vi "Get User Filename and Path.vi"(8 "error in (no error)":errorcluster) -> (0 "error out":errorcluster, 2 "TXT File Path":path, 3 "CSV File Path":path)   [LabVIEW 2021]
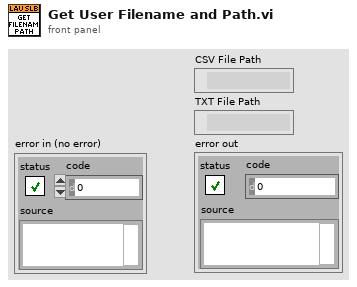
[diagram p1: front panel]
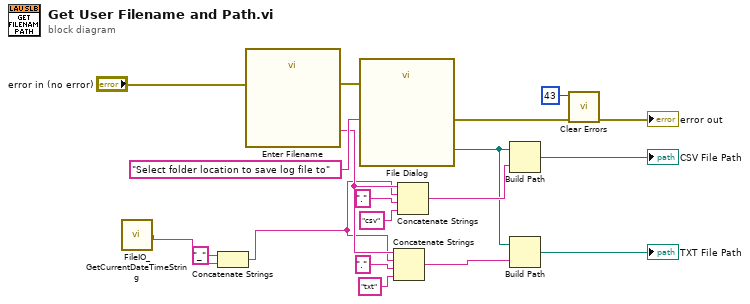
[diagram p0: block diagram]
diagram:
  n1 = call "FileIO_GetCurrentDateTimeString.vi"() -> ("Date/Time String"=w3:string)  [unwired: 14 in, 1 out]
  n2 = Concatenate Strings("_" ("string"), w3) -> (w1:string)
  n3 = call "Enter Filename"("error in (no error)"="error in (no error)") -> ("Filename"=w12:string, "error out"=w19:errorcluster)  [unwired: 16 in, 1 out]
  n4 = call "File Dialog"("prompt"="Select folder location to save log file to", "error in"=w19) -> ("selected path"=w13:path, "error out"=w10:errorcluster)  [unwired: 10 in, 2 out]
  n5 = Concatenate Strings(w12, w1, "." ("string"), "txt" ("string")) -> (w14:string)
  n6 = Concatenate Strings(w12, w1, "." ("string"), "csv" ("string")) -> (w17:string)
  n7 = Build Path(base path=w13, name or relative path=w17) -> (appended path=→"CSV File Path":path)
  n8 = Build Path(base path=w13, name or relative path=w14) -> (appended path=→"TXT File Path":path)
  n9 = call <vilib>:"Clear Errors.vi"("error in (no error)"=w10, "specific error code to clear (0: all)"=43) -> ("error out"=→"error out":errorcluster)  [unwired: 4 in, 1 out]
